vi "Reconfigure.vi"(8 "error in (no error)":errorcluster, 10 "navX - Interface Update in":refnum<class "navX - Interface.lvclass">, 11 "navX - Interface in":refnum<class "navX - Interface.lvclass">) -> (0 "error out":errorcluster, 3 "navX - Interface out":refnum<class "navX - Interface.lvclass">)   [LabVIEW 2015, in "navX Library v3.lvlib" / "navX - Interface.lvclass"]
uses:
  navX - Interface.lvclass
  navX - Interface.lvclass/navX - Interface.ctl
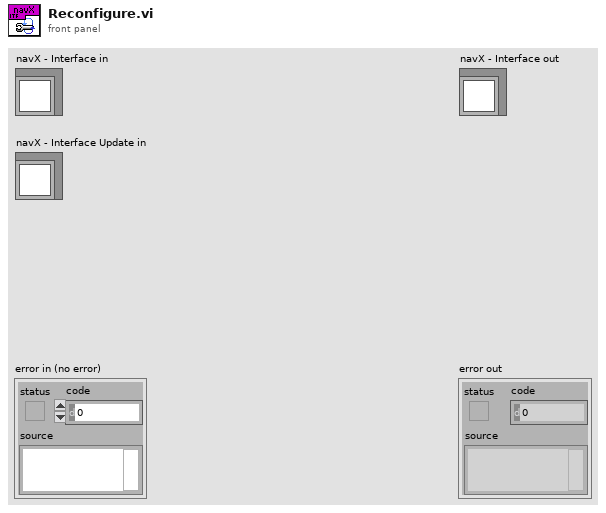
[diagram p1: front panel]
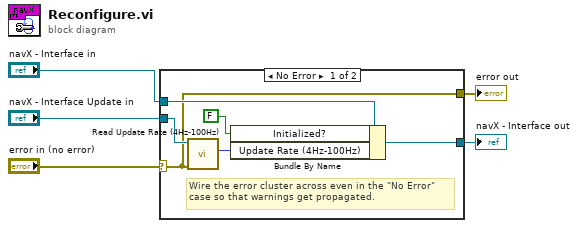
[diagram p0: block diagram]
diagram:
  n1 = case shown="No Error" "error in (no error)" {
    selector: "error in (no error)" -> [w7 w13]
    tunnel: [w7 w13] -> w4
    tunnel: [w10 w12] -> w2
    tunnel: "navX - Interface in" -> [w11 w12]
    tunnel: "navX - Interface Update in" -> [w8 _]
    frame No Error {
      # "Wire the error cluster across even in the \"No Error\"\ncase so that warnings get propagated."
      n2 = call "Read Update Rate (4Hz-100Hz).vi"("error in (no error)"=w7, "navX - Interface in"=w8) -> ("Update Rate (4Hz-100Hz)"=w6:u8)  [unwired: 7 in, 2 out]
      n3 = Bundle By Name(cluster=w11, "Initialized?"=FALSE, "Update Rate (4Hz-100Hz)"=w6) -> (w10:refnum<class "navX - Interface.lvclass">)
    }
    frame Error {
    }
  }
  "error out" <- w4
  "navX - Interface out" <- w2
